vi "3waySwitchSingle-Mod - Copy.vi"() -> ()   [LabVIEW 2012]
panel:
  out "Boolean 2":bool
  out "Boolean":bool
  in  "STOP":bool
  in  "GO":bool
  out "number":u32
  in  "stop":bool
  in  "ON":bool
  in  "OFF":bool
  # "Christian Altenbach, May 2005, caltenba@ucla.edu\nModified by Daniel Hartmann, 28 Feb, 2012"
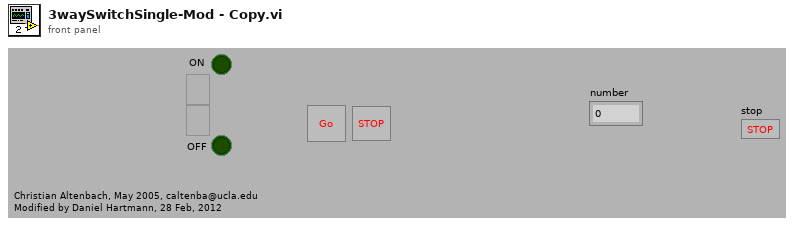
[diagram p1: front panel]
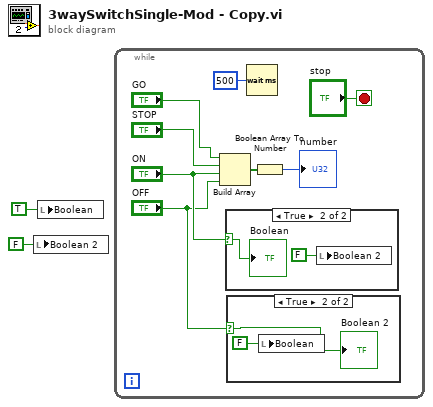
[diagram p0: block diagram]
diagram:
  n1 = local write "Boolean 2"(FALSE ("Boolean 2")) -> ()
  n2 = local write "Boolean"(TRUE ("Boolean")) -> ()
  n3 = while {
    stop <- "stop" stop-if-true
    n4 = Build Array("GO", "STOP", "ON", "OFF") -> (w8:bool[])
    n5 = case shown="True" "ON" {
      selector: "ON" -> [_ w14]
      frame False {
      }
      frame True {
        n6 = local write "Boolean 2"(FALSE ("Boolean 2")) -> ()
        "Boolean" <- w14
      }
    }
    n7 = case shown="True" "OFF" {
      selector: "OFF" -> [_ w11]
      frame False {
      }
      frame True {
        n8 = local write "Boolean"(FALSE ("Boolean")) -> ()
        "Boolean 2" <- w11
      }
    }
    n9 = Wait (ms)(milliseconds to wait=u32 500) -> ()  [unwired: 1 out]
    n10 = Boolean Array To Number(Boolean array=w8) -> (number=→"number":u32)
  }
